vi "态-路径未实现.vi"(5 "检查动作?":bool, 7 "枚举-错误类型":T1, 8 "错误输入":errorcluster) -> (0 "错误输出":errorcluster, 3 "枚举-错误类型 o":T1, 6 "输入":cluster{"路径枚举名":string})   [LabVIEW 2017]
panel:
  # "1. 修改本VI的动作类型输出值\n2. 定义输入输出类型, 并连到接线板底端"
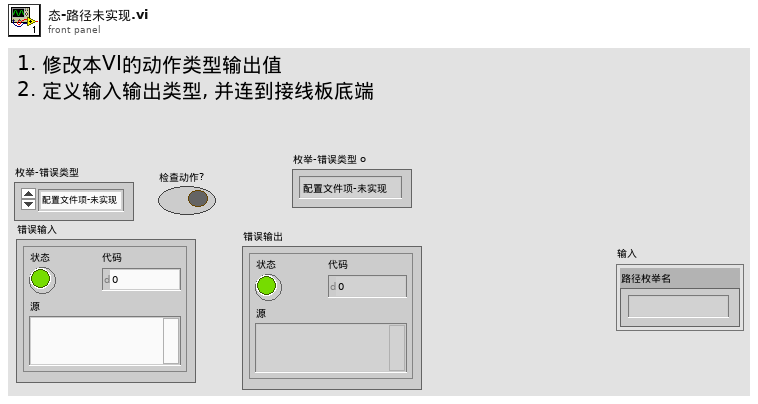
[diagram p1: front panel]
types:
  T1 = typedef "调试与报错.lvlib/枚举-错误类型.ctl" = enum16{"配置文件项-未实现", "路径-未实现"}
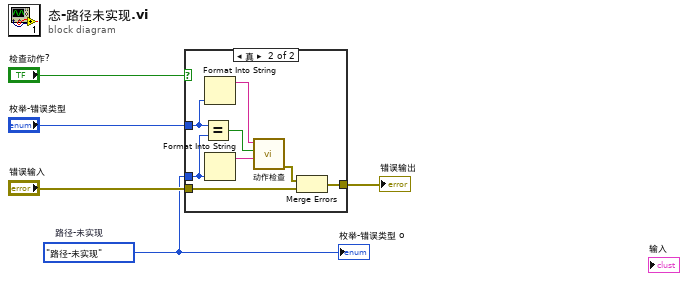
[diagram p0: block diagram]
diagram:
  w2 = 枚举-错误类型."路径-未实现"  # 路径-未实现
  n1 = case shown="真" "检查动作?" {
    tunnel: "错误输入" -> [w6 w14]
    tunnel: [w6 w13] -> w4
    tunnel: "枚举-错误类型" -> [_ w11]
    tunnel: w2 -> [_ w7]
    frame False {
    }
    frame True {
      n2 = Equal?(x=w11, y=w7) -> (x = y?=w12:bool)
      n3 = Format Into String(w11) -> (resulting string=w10:string)  [unwired: 3 in, 1 out]
      n4 = Format Into String(w7) -> (resulting string=w9:string)  [unwired: 3 in, 1 out]
      n5 = call "动作检查.vi"("需要动作"=w9, "动作枚举类型匹配?"=w12, "传入动作"=w10) -> ("输出簇"=w8:errorcluster)  [unwired: 8 in]
      n6 = Merge Errors(w8, w14) -> (w13:errorcluster)
    }
  }
  "错误输出" <- w4
  "枚举-错误类型 o" <- w2
